vi "Write Data.vi"(8 "error in (no error)":errorcluster, 9 "Publication Time":timestamp, 10 "Value":variant, 11 "PersistToDiskTransport In":refnum<class "PersistToDiskTransport.lvclass">) -> (0 "error out":errorcluster, 3 "PersistToDiskTransport Out":refnum<class "PersistToDiskTransport.lvclass">)   [LabVIEW 2020, in "PersistToDiskTransport.lvclass"]
doc: "<License>\nCopyright © 2017 Composed Systems, LLC | All rights reserved\nwww.composed.io\n\nAuthor: Ethan Stern <ethan.stern@composed.io>\n\nThis software is provided \"AS IS\" WITHOUT WARRANTIES, either express or implied, AND IS FOR EDUCATIONAL PURPOSES ONLY.\n</License>"
uses:
  <vilib>/gpm_packages/@cs/transport/Source/Concrete/PersistToDiskTransport/PersistToDiskTransport.lvclass
  <vilib>/gpm_packages/@cs/transport/Source/Concrete/PersistToDiskTransport/PersistToDiskTransport.lvclass/PersistToDiskTransport.ctl
  <vilib>/Utility/error.llb/Error Cluster From Error Code.vi
  <vilib>/gpm_packages/@cs/variant/Source/Format Type String.vi
  <vilib>/ErrorRing/Error Ring.xnode
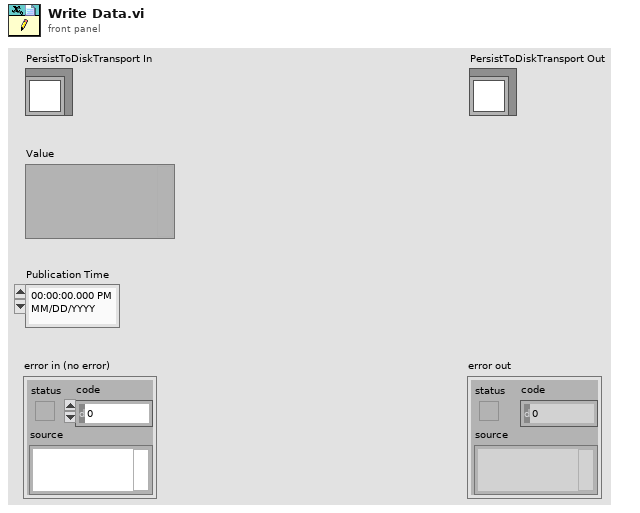
[diagram p1: front panel]
types:
  T1 = cluster{"Datum Name":string, "type string":i16[], "data string":string, "Publication Time":timestamp}
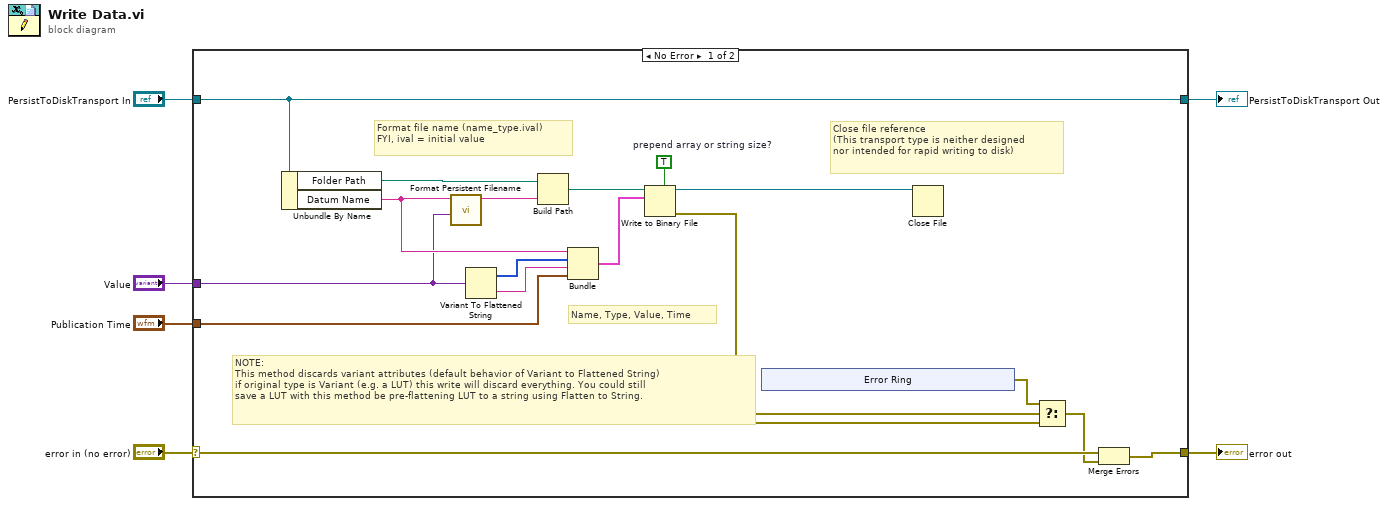
[diagram p0: block diagram]
diagram:
  n1 = case shown="No Error" "error in (no error)" {
    selector: "error in (no error)" -> [w11 w29]
    tunnel: "PersistToDiskTransport In" -> [w10 w30]
    tunnel: [w23 w29] -> w5
    tunnel: "Publication Time" -> [w16 _]
    tunnel: "Value" -> [w12 _]
    tunnel: [w10 w30] -> w1
    frame No Error {
      w20 = TRUE  # prepend array or string size?
      # "Close file reference\n(This transport type is neither designed\nnor intended for rapid writing to disk)"
      # "Name, Type, Value, Time"
      # "NOTE:\nThis method discards variant attributes (default behavior of Variant to Flattened String)\nif original type is Variant (e.g. a LUT) this write will discard everything. You could still\nsave a LUT with this method be pre-flattening LUT to a string using Flatten to String."
      # "Format file name (name_type.ival)\nFYI, ival = initial value"
      n2 = Unbundle By Name(w10) -> ("Folder Path"=w22:path, "Datum Name"=w17:string)
      n3 = call <vilib>:"Format Persistent Filename.vi"("Datum Type"=w12, "Datum Name"=w17) -> ("Filename"=w14:string)  [unwired: 9 in]
      n4 = Variant To Flattened String(Variant=w12) -> (data string=w18:string, 1:w19:i16[])
      n5 = Build Path(base path=w22, name or relative path=w14) -> (appended path=w21:path)
      n6 = Bundle("Datum Name"=w17, "type string"=w19, "data string"=w18, "Publication Time"=w16) -> (w15:T1)  [unwired: 1 in]
      n7 = Write to Binary File(file (use dialog)=w21, data=w15, 5:w20) -> (refnum out=w13:refnum<file>, error out=w9:errorcluster)  [unwired: 3 in, 1 out]
      n8 = xnode "Error Ring"() -> ("error out"=w7:errorcluster)
      n9 = Close File(refnum=w13) -> ()  [unwired: 1 in, 2 out]
      n10 = Select(t=w7, s=w9, f=w9) -> (s? t:f=w8:errorcluster)
      n11 = Merge Errors(w11, w8) -> (w23:errorcluster)
    }
    frame Error {
    }
  }
  "error out" <- w5
  "PersistToDiskTransport Out" <- w1
